vi "Test Connection.vi"() -> ()   [LabVIEW 2019, in "Logger.lvclass"]
uses:
  Logger.lvclass
  ObjData.ctl
  ObjType.ctl
  SignalData.ctl
  EventData.ctl
  TypeDef/AlarmType.ctl
  Database_Postgress_class/Database_Postgress.lvclass
  D:/GIT H4000/H4000/src/DatabaseInterface_class/DatabaseInterface.lvclass
  Database_Postgress_class/Connection Info.ctl
  Logger.lvclass/Logger.ctl
  DatabaseInterface_class/DatabaseInterface.lvclass
panel:
  in  "Events 2":T1[](array[typedef])=[{"obj_tag"="o_tag_1", "event_tag"="o_tag_1_di", "Description"="dsfsadf", "ALARM TYPE"=enum."Alarm", "Value DBL"=234.0, "Value INT"=23423, "Value STR"="xfddf", "Time Stamp"=timestamp(3831350232.4442434 s since 1904-01-01)}]
  in  "sig":T3[](array[typedef])=[{"Value"=1.0, "SignalTag"="s_tag_1", "ObjTag"="o_tag_1", "Desc"="dfs", "Time Stamp"=timestamp(3831177088.422016 s since 1904-01-01)}, {"Value"=2.0, "SignalTag"="s_tag_1", "ObjTag"="o_tag_1", "Desc"="dfas", "Time Stamp"=timestamp(3831263490.641324 s since 1904-01-01)}, {"Value"=3.0, "SignalTag"="s_tag_2", "ObjTag"="o_tag_1", "Desc"="dfsd", "Time Stamp"=timestamp(3830140293.1623626 s since 1904-01-01)}]
  in  "Array":T4[](array[typedef])=[{"object_tag"="o_tag", "parent_tag"="p_tag", "object_type"=enum."Device", "description"="Тестовый обект"}]
  out "error out":errorcluster
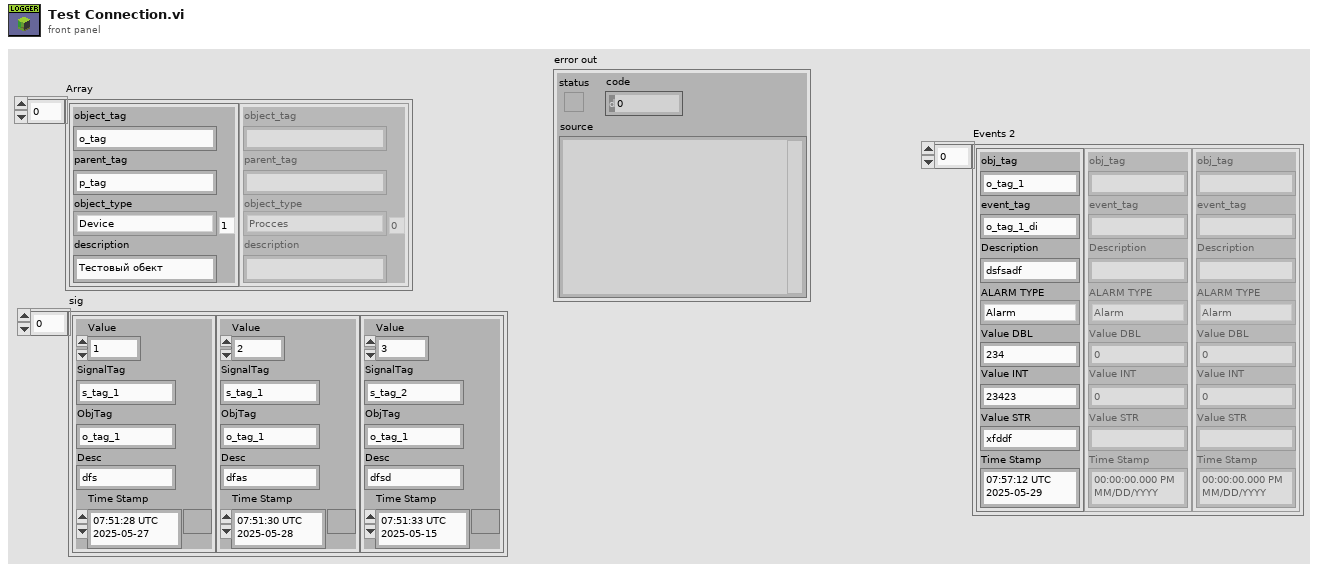
[diagram p1: front panel]
types:
  T1 = typedef "EventData.ctl" = cluster{"obj_tag":string, "event_tag":string, "Description":string, "ALARM TYPE":T2, "Value DBL":dbl, "Value INT":i32, "Value STR":string, "Time Stamp":timestamp}
  T2 = typedef "AlarmType.ctl" = enum16{"Normal", "Warning", "Alarm"}
  T3 = typedef "Logger.lvclass/SignalData.ctl" = cluster{"Value":dbl, "SignalTag":string, "ObjTag":string, "Desc":string, "Time Stamp":timestamp}
  T4 = typedef "Logger.lvclass/ObjData.ctl" = cluster{"object_tag":string, "parent_tag":string, "object_type":T5, "description":string}
  T5 = typedef "Logger.lvclass/ObjType.ctl" = enum16{"Procces", "Device", "Signal", "DI", "DO", "DA", "AI", "AO", "AA"}
  T6 = typedef "DatabaseInterface.lvclass/Connection Info.ctl" = cluster{"IP_Address":string, "Port":u16, "Timeout":i32, "User":string, "Password":string, "Database":string}
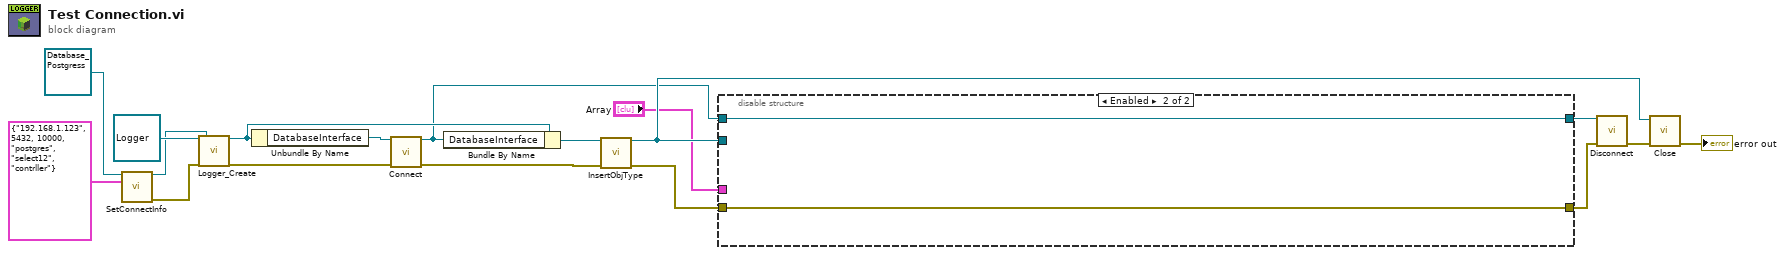
[diagram p0: block diagram]
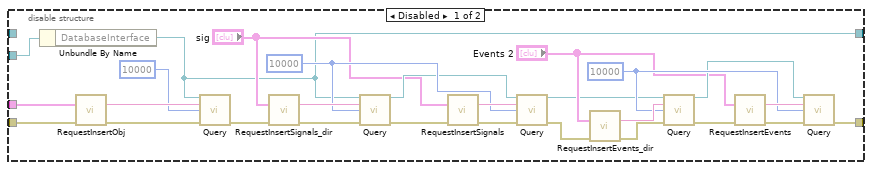
[diagram p2: hidden frame]
diagram:
  n1 = call-dynamic "SetConnectInfo.vi"("reference in"=refnum<class "Database_Postgress.lvclass"> refnum, "Connection Info"=T6 {"IP_Address"="192.168.1.123", "Port"=5432, "Timeout"=10000, "User"="postgres", "Password"="select12", "Database"="contrller"}) -> ("reference out"=w13:refnum<class "Database_Postgress.lvclass">, "error out"=w15:errorcluster)  [unwired: 12 in]
  n2 = call "Logger_Create.vi"("reference in"=refnum<class "Logger.lvclass"> refnum, "error in (no error)"=w15, "DatabaseInterface"=w13) -> ("reference out"=w9:refnum<class "Logger.lvclass">, "error out"=w11:errorcluster)  [unwired: 15 in]
  n3 = Unbundle By Name(w9) -> ("DatabaseInterface"=w12:refnum<class "DatabaseInterface.lvclass">)
  n4 = call-dynamic "Connect.vi"("reference in"=w12, "error in (no error)"=w11) -> ("reference out"=w1:refnum<class "DatabaseInterface.lvclass">, "error out"=w8:errorcluster)  [unwired: 12 in]
  n5 = Bundle By Name(cluster=w9, "DatabaseInterface"=w1) -> (w7:refnum<class "Logger.lvclass">)
  n6 = call "InsertObjType.vi"("reference in"=w7, "error in (no error)"=w8) -> ("reference out"=w6:refnum<class "Logger.lvclass">, "error out"=w4:errorcluster)  [unwired: 11 in, 1 out]
  n7 = disable-structure shown="Enabled" {
    disable-tunnel: w6 -> [w45 _]
    disable-tunnel: "Array" -> [w41 _]
    disable-tunnel: w4 -> [w40 w47]
    disable-tunnel: [w31 w46] -> w3
    disable-tunnel: [w19 w47] -> w2
    disable-tunnel: w1 -> [_ w46]
    frame Disabled {
      w26 = 10000 ("Timeout")
      w36 = 10000 ("Timeout")
      n8 = Unbundle By Name(w45) -> ("DatabaseInterface"=w31:refnum<class "DatabaseInterface.lvclass">)
      n9 = call "RequestInsertObj.vi"("Array"=w41, "error in (no error)"=w40) -> ("request"=w43:string, "error out"=w44:errorcluster)  [unwired: 12 in]
      n10 = call-dynamic "Query.vi"("reference in"=w31, "Query"=w43, "Timeout"=10000, "error in (no error)"=w44) -> ("error out"=w30:errorcluster)  [unwired: 9 in, 2 out]
      n11 = call "RequestInsertSignals_dir.vi"("Signals"="sig", "error in (no error)"=w30) -> ("request"=w37:string, "error out"=w34:errorcluster)  [unwired: 12 in]
      n12 = call-dynamic "Query.vi"("reference in"=w31, "Query"=w37, "Timeout"=w36, "error in (no error)"=w34) -> ("reference out"=w35:refnum<class "DatabaseInterface.lvclass">, "error out"=w33:errorcluster)  [unwired: 9 in, 1 out]
      n13 = call "RequestInsertSignals.vi"("Events"="sig", "error in (no error)"=w33) -> ("request"=w38:string, "error out"=w39:errorcluster)  [unwired: 12 in]
      n14 = call-dynamic "Query.vi"("reference in"=w35, "Query"=w38, "Timeout"=w36, "error in (no error)"=w39) -> ("reference out"=w21:refnum<class "DatabaseInterface.lvclass">, "error out"=w20:errorcluster)  [unwired: 9 in, 1 out]
      n15 = call "RequestInsertEvents_dir.vi"("Events"="Events 2", "error in (no error)"=w20) -> ("request"=w27:string, "error out"=w24:errorcluster)  [unwired: 12 in]
      n16 = call-dynamic "Query.vi"("reference in"=w21, "Query"=w27, "Timeout"=w26, "error in (no error)"=w24) -> ("reference out"=w25:refnum<class "DatabaseInterface.lvclass">, "error out"=w23:errorcluster)  [unwired: 9 in, 1 out]
      n17 = call "RequestInsertEvents.vi"("Events"="Events 2", "error in (no error)"=w23) -> ("request"=w28:string, "error out"=w29:errorcluster)  [unwired: 12 in]
      n18 = call-dynamic "Query.vi"("reference in"=w25, "Query"=w28, "Timeout"=w26, "error in (no error)"=w29) -> ("error out"=w19:errorcluster)  [unwired: 9 in, 2 out]
    }
    frame Enabled {
    }
  }
  n19 = call-dynamic "Disconnect.vi"("reference in"=w3, "error in (no error)"=w2) -> ("error out"=w10:errorcluster)  [unwired: 12 in, 1 out]
  n20 = call "Close.vi"("error in (no error)"=w10, "Logger in"=w6) -> ("error out"=→"error out":errorcluster)  [unwired: 8 in, 1 out]
